vi "Launch Root Actor_Actor_Generates Actor Traces.vi"() -> ()   [LabVIEW 2020]
uses:
  ActorFramework/Actor/Actor.lvclass
  ActorFramework/Message Enqueuer/Message Enqueuer.lvclass/Message Enqueuer.ctl
  ActorFramework/Message Enqueuer/Enqueue.vi
  ActorFramework/Stop Msg/Stop Msg.lvclass
  C:/justACS/Actor Framework/Core/ActorFramework/Message/Message.lvclass
  <vilib>/Utility/LVClass/Get LV Class Name.vi
  ActorFramework/tracing/Trace Generation/Generate Trace for Message.vi
  ActorFramework/Message Priority Queue/Priority Enqueue.vi
  <vilib>/addons/_JKI Toolkits/Caraya/classes/Assert/Assert Equal Value_Variant.vi
  <vilib>/addons/_JKI Toolkits/Caraya/classes/Test/Test.lvclass
  <vilib>/addons/_JKI Toolkits/Caraya/classes/Assert/Assert.lvclass
  Test Harness/AF Trace Queue/AF Trace Queue.lvclass
panel:
  out "error out":errorcluster
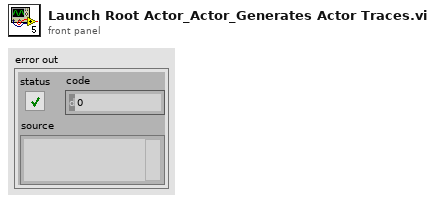
[diagram p1: front panel]
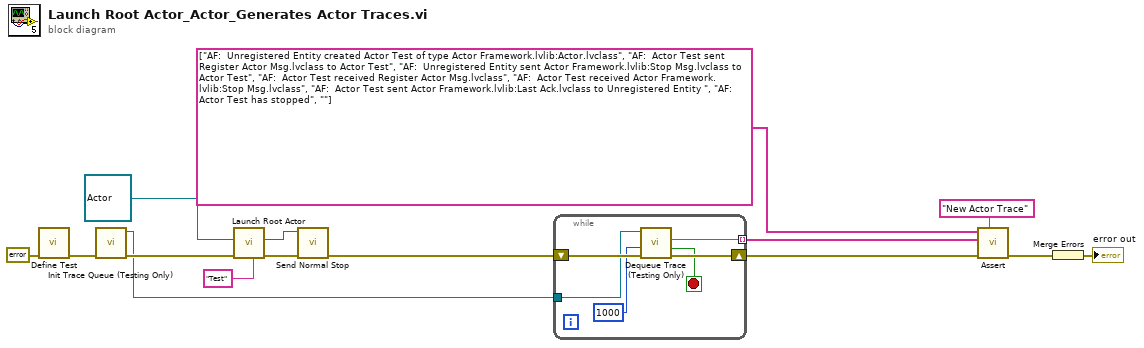
[diagram p0: block diagram]
diagram:
  n1 = call <vilib>:"Define Test.vi"("error in (no error)"=errorcluster {"status"=FALSE, "code"=0, "source"=""}) -> ("error out"=w14:errorcluster)  [unwired: 9 in, 1 out]
  n2 = call "Init Trace Queue (Testing Only).vi"("error in (no error)"=w14) -> ("error out"=w11:errorcluster, "AF Trace Queue out"=w6:refnum<class "AF Trace Queue.lvclass">)  [unwired: 9 in]
  n3 = call "Launch Root Actor.vi"("Debug Alias"="Test", "error in (no error)"=w11, "Actor"=refnum<class "Actor.lvclass"> refnum ("Actor Framework:Actor")) -> ("error out"=w10:errorcluster, "Actor's Enqueuer"=w8:refnum<class "Message Enqueuer.lvclass">)  [unwired: 7 in]
  n4 = call "Send Normal Stop.vi"("error in (no error)"=w10, "Message Enqueuer"=w8) -> ("error out"=w9:errorcluster)  [unwired: 9 in]
  n5 = while {
    tunnel: w6 -> [w20]
    shift-right: [w19] -> w4
    shift-left: w9 -> [w21]
    tunnel: [w16] -> w2 mode=indexing
    stop <- w17 stop-if-true
    n6 = call "Dequeue Trace (Testing Only).vi"("error in (no error)"=w21, "timeout in ms (-1)"=1000, "AF Trace Queue in"=w20) -> ("error out"=w19:errorcluster, "timed out?"=w17:bool, "Trace String"=w16:string)  [unwired: 5 in, 1 out]
  }
  n7 = call-poly <vilib>:"Assert.vi"("Label"="New Actor Trace" ("Label (VI Title)"), "error in (no error)"=w4, "Y"=w2, "X"=string[] ["AF:  Unregistered Entity created Actor Test of type Actor Framework.lvlib:Actor.lvclass", "AF:  Actor Test sent Register Actor Msg.lvclass to Actor Test", "AF:  Unregistered Entity sent Actor Framework.lvlib:Stop Msg.lvclass to Actor Test", "AF:  Actor Test received Register Actor Msg.lvclass", "AF:  Actor Test received Actor Framework.lvlib:Stop Msg.lvclass", "AF:  Actor Test sent Actor Framework.lvlib:Last Ack.lvclass to Unregistered Entity ", "AF:  Actor Test has stopped", ""] ("Array")) -> ("error out"=w3:errorcluster)  [unwired: 6 in, 1 out]
  n8 = Merge Errors(w3) -> (→"error out":errorcluster)
